vi "Add_Update_Values_sub.vi"(5 "Raw data Filename column name":string, 6 "Edit all Rows?":bool, 7 "Value  Constant?":bool, 8 "Selected Rows":i32[](array[numeric]), 9 "New Values In":string[][](array[string]), 10 "New Chs In":string[](array[string])=[""], 11 "Filename":path) -> (1 "Edit Info":string[][](array[string]))   [LabVIEW 2010]
uses:
  Globals/Constants_global.vi
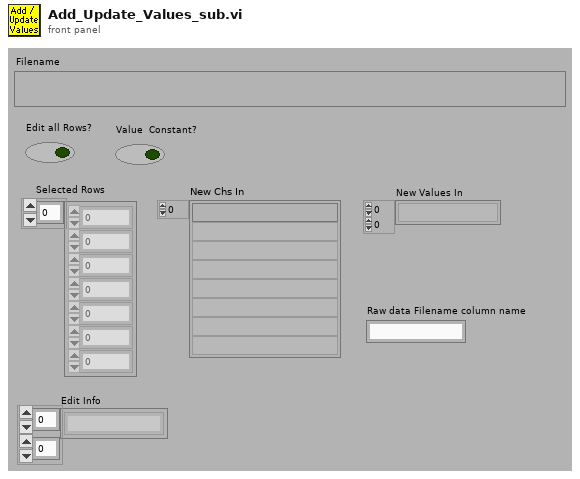
[diagram p1: front panel]
types:
  T1 = enum16{"read/write", "read-only", "write-only", "write-only (truncate)"}
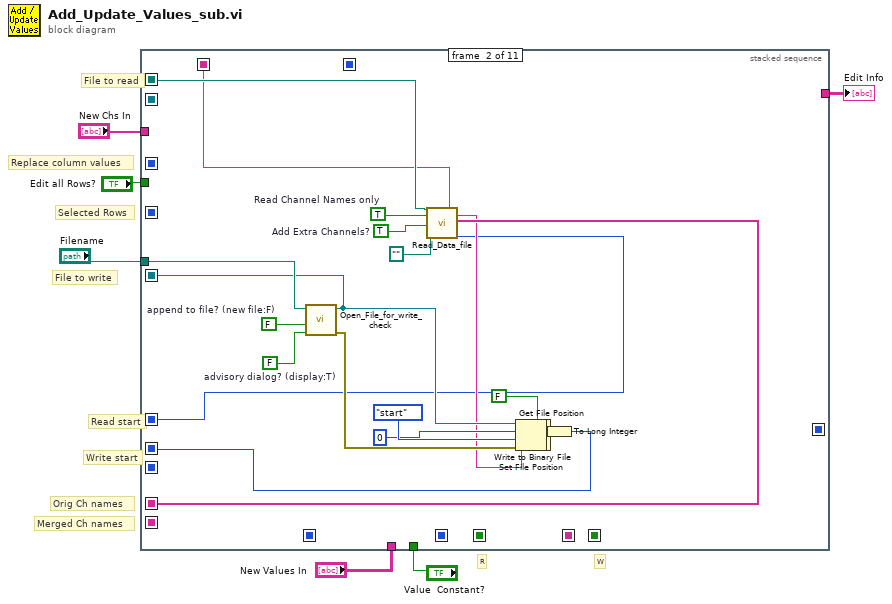
[diagram p0: block diagram]
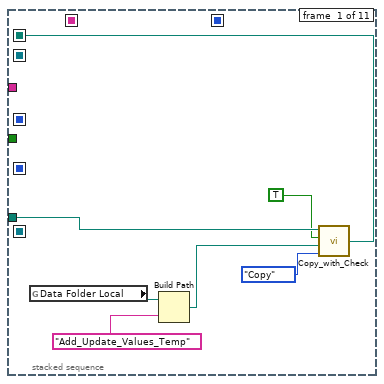
[diagram p2: hidden frame]
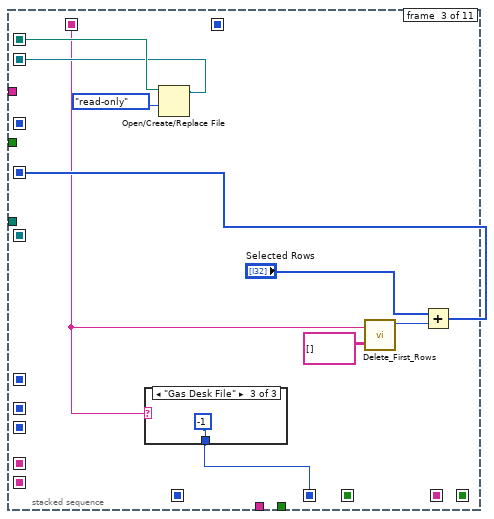
[diagram p3: hidden frame]
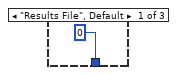
[diagram p4: hidden frame]
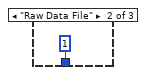
[diagram p5: hidden frame]
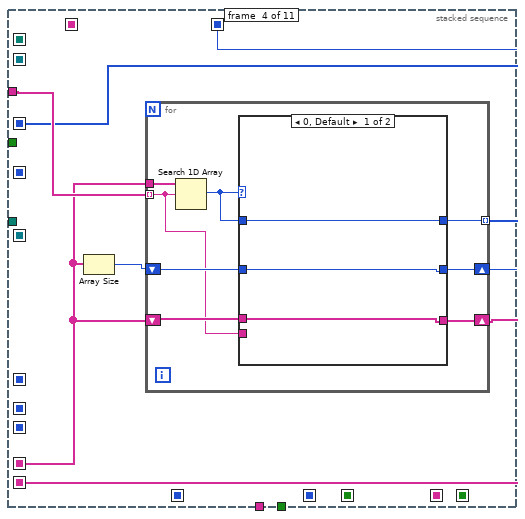
[diagram p6: hidden frame]
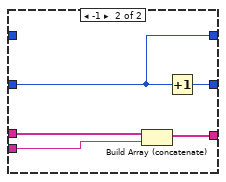
[diagram p7: hidden frame]
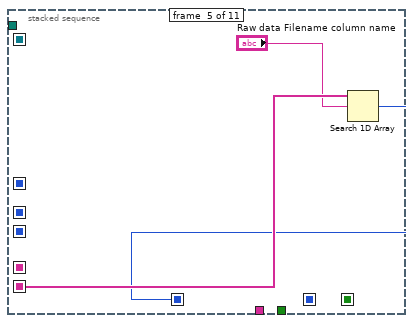
[diagram p8: hidden frame]
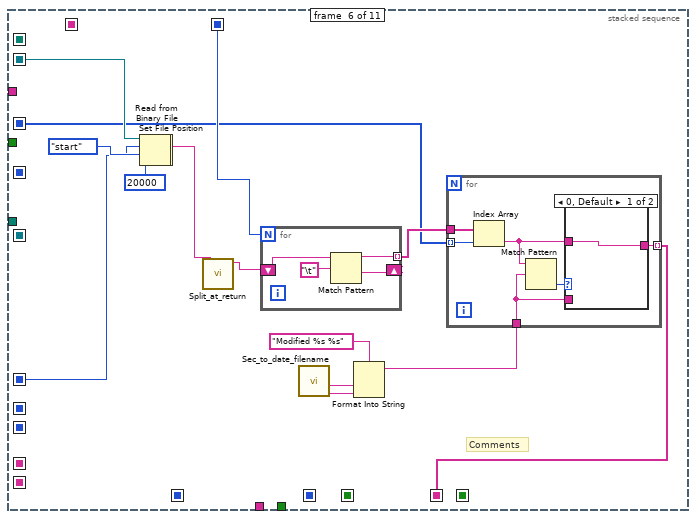
[diagram p9: hidden frame]
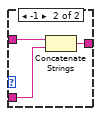
[diagram p10: hidden frame]
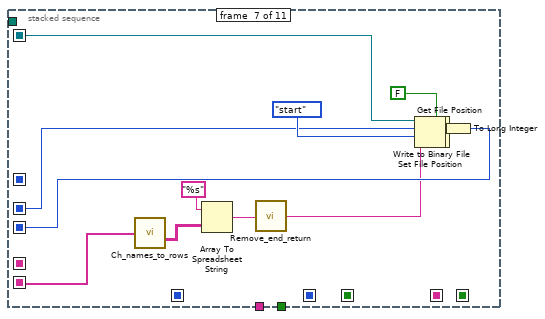
[diagram p11: hidden frame]
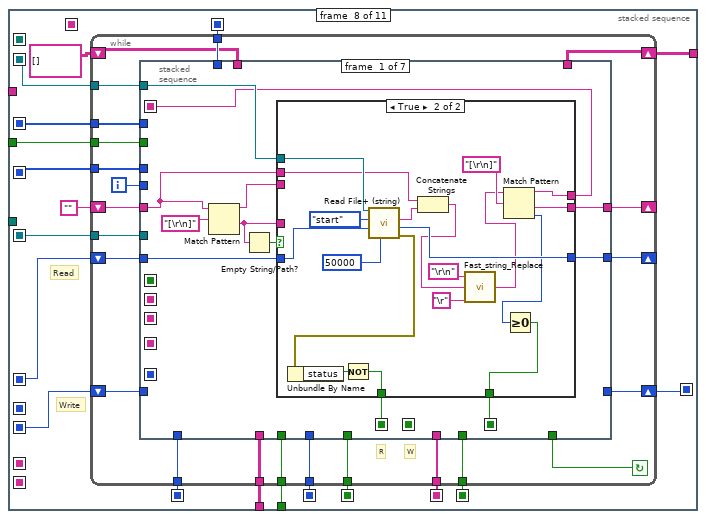
[diagram p12: hidden frame]
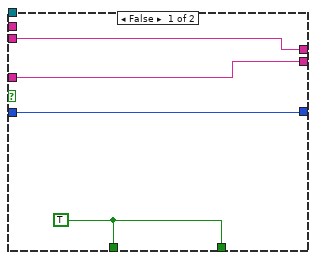
[diagram p13: hidden frame]
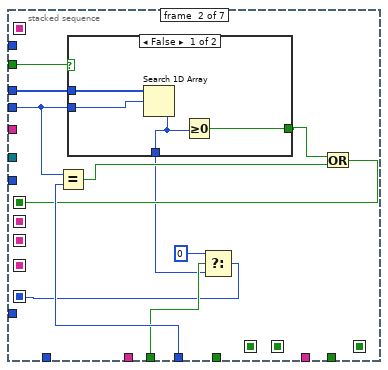
[diagram p14: hidden frame]
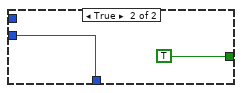
[diagram p15: hidden frame]
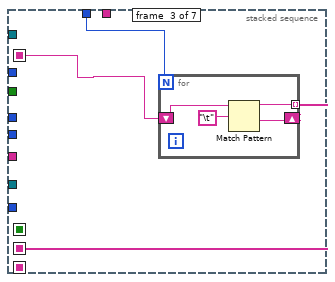
[diagram p16: hidden frame]
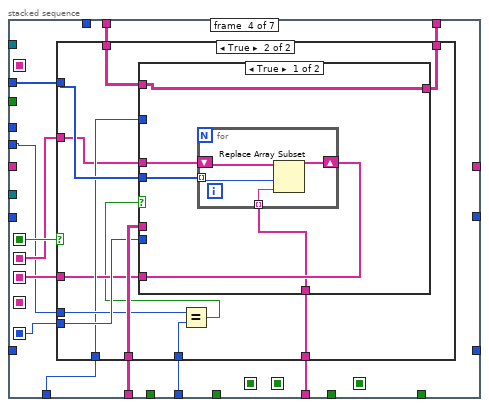
[diagram p17: hidden frame]
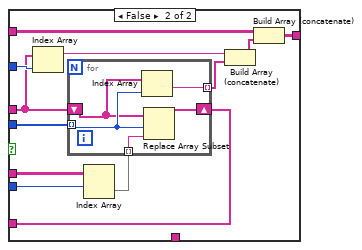
[diagram p19: hidden frame]
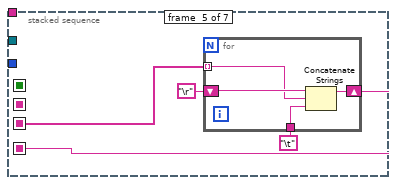
[diagram p20: hidden frame]
diagram:
  # "File to read"
  # "File to write"
  # "Merged Ch names"
  # "Orig Ch names"
  # "Replace column values"
  # "Selected Rows"
  # "Read start"
  # "Write start"
  # "W"
  # "R"
  n1 = stacked-sequence {
    seq-local: [_ _ w39 _ _ _ _ _ _ _ _] -> [_ _ _ _ _ w86 _ w129 _ w306 _]
    seq-local: [_ w22 _ _ _ _ _ _ _ _ _] -> [_ _ _ _ _ w85 _ w131 _ _ _]
    seq-local: [_ _ _ _ _ _ _ w135 _ _ _] -> [_ _ _ _ _ _ _ _ _ _ w310]
    seq-local: [_ _ _ _ _ _ _ w134 _ _ _] -> [_ _ _ _ _ _ _ _ _ _ w312]
    seq-local: [_ _ _ _ _ _ _ w133 _ _ _] -> [_ _ _ _ _ _ _ _ w303 _ _]
    seq-local: [_ _ w42 _ _ _ _ _ _ _ _] -> [_ _ _ _ _ _ _ w132 _ _ _]
    seq-local: [_ w23 _ _ _ _ _ _ _ _ _] -> [_ _ _ _ _ _ w111 _ _ _ _]
    seq-local: [_ w33 _ _ _ _ _ _ _ _ _] -> [_ _ _ w50 _ _ _ _ _ _ _]
    seq-local: [_ _ _ w51 _ _ _ _ _ _ _] -> [_ _ _ _ _ w80 _ w127 _ _ _]
    seq-local: [_ w25 _ _ _ _ _ _ _ _ _] -> [_ _ _ _ _ _ w112 w130 w301 w304 _]
    seq-local: [_ _ _ w49 _ _ _ _ _ _ _] -> [_ _ _ _ _ w88 _ w128 _ _ _]
    seq-local: [_ _ _ w48 _ _ _ _ _ _ _] -> [_ _ _ _ w72 _ w115 _ _ _ _]
    seq-local: [w8 _ _ _ _ _ _ _ _ _ _] -> [_ w32 w40 _ _ _ _ _ _ _ w308]
    seq-local: [_ _ _ _ _ _ w110 _ _ _ _] -> [_ _ _ _ _ _ _ w126 _ _ _]
    seq-local: [_ w21 _ _ _ _ _ _ _ _ _] -> [_ _ w37 _ _ _ _ _ _ _ _]
    seq-local: [_ _ _ _ _ w76 _ _ _ _ _] -> [_ _ _ _ _ _ _ w121 _ _ _]
    seq-local: [_ _ w38 _ _ _ _ _ _ _ _] -> [_ _ _ _ _ _ _ w122 _ _ _]
    seq-local: [_ _ _ _ w71 _ _ _ _ _ _] -> [_ _ _ _ _ _ _ w120 _ _ _]
    tunnel: "Filename" -> [w10 w26 _ _ _ _ _ _ _ _ w309]
    tunnel: "New Chs In" -> [_ _ _ w53 _ _ _ _ _ _ _]
    tunnel: "Edit all Rows?" -> [_ _ _ _ _ _ _ w125 _ _ _]
    tunnel: "New Values In" -> [_ _ _ _ _ _ _ w124 _ _ _]
    tunnel: "Value  Constant?" -> [_ _ _ _ _ _ _ w123 _ _ _]
    tunnel: [_ _ _ _ _ _ _ w118 _ _ _] -> w1
    frame #0 {
      n2 = global read "Constants_global.vi" "Data Folder Local"() -> (w12:path)
      n3 = Build Path(base path=w12, name or relative path="Add_Update_Values_Temp") -> (appended path=w11:path)
      n4 = call "Copy_with_Check.vi"("Mode"=enum16{"Move", "Copy"}."Copy", "Target Path"=w11, "Variable Target?"=TRUE, "Source Path"=w10) -> ("Pathname Out"=w8:path)
    }
    frame #1 {
      w14 = TRUE  # Add Extra Channels?
      w30 = FALSE  # advisory dialog? (display:T)
      w31 = FALSE  # append to file? (new file:F)
      w34 = TRUE  # Read Channel Names only
      n5 = call "Open_File_for_write_check.vi"("advisory dialog? (display:T)"=w30, "append to file? (new file:F)"=w31, "file path"=w26) -> ("error out"=w27:errorcluster, "refnum"=w25:refnum<file>)  [unwired: 7 out]
      n6 = call "Read_Data_file.vi"("Results file"=w32, "Read Channel Names only"=w34, "Add Extra Channels?"=w14, "Template File"=path "") -> ("Filetype"=w21:string, "String Before"=w24:string, "Ch names Out"=w33:string[], "mark after read (chars.)"=w22:i32)  [unwired: 1 in, 11 out]
      n7 = Set File Position(offset (in bytes) (0)=0 ("pos offset (0)"), refnum=w25, from (0:start)=enum16{"start", "end", "current"}."start" ("pos mode (0:2)"), error in=w27) -> (refnum out=w20:refnum<file>, error out=w19:errorcluster)
      n8 = Write to Binary File(file (use dialog)=w20, data=w24, error in=w19, 5:FALSE ("prepend array or string size? (T)")) -> (refnum out=w18:refnum<file>, error out=w17:errorcluster)  [unwired: 3 out]
      n9 = Get File Position(4:w17, 7:w18) -> (2:w16:i64)  [unwired: 2 out]
      n10 = To Long Integer(number=w16) -> (32bit integer=w23:i32)
    }
    frame #2 {
      n11 = case shown="\"Gas Desk File\"" w37 {
        tunnel: [0 ("Comments Row Number") 1 ("Comments Row Number") -1 ("Comments Row Number")] -> w38
        frame "Results File", Default {
        }
        frame "Raw Data File" {
        }
        frame "Gas Desk File" {
        }
      }
      n12 = Open/Create/Replace File(file path (use dialog)=w40, access (0:read/write)=T1."read-only" ("open mode (0)")) -> (refnum out=w39:refnum<file>)  [unwired: 1 in, 5 out]
      n13 = call "Delete_First_Rows.vi"("Data In"=string[][] [], "File Type"=w37) -> ("Rows removed"=w44:i32)  [unwired: 1 out]
      n14 = Add(x="Selected Rows", y=w44) -> (x+y=w42:i32[])
    }
    frame #3 {
      n15 = Array Size(array=w50) -> (size(s)=w52:i32)
      n16 = for {
        tunnel: w50 -> [w61]
        tunnel: w53 -> [w54] mode=indexing
        shift-right: [w60] -> w49
        shift-left: w52 -> [w59]
        tunnel: [w58] -> w51 mode=indexing
        shift-right: [w55] -> w48
        shift-left: w50 -> [w56]
        n17 = Search 1D Array(1D array=w61, element=w54) -> (index of element=w57:i32)  [unwired: 1 out]
        n18 = case shown="0, Default" w57 {
          tunnel: [w63 w69] -> w60
          tunnel: w59 -> [w63 w68]
          tunnel: [w64 w68] -> w58
          tunnel: w57 -> [w64 _]
          tunnel: w56 -> [w62 w67]
          tunnel: [w62 w66] -> w55
          tunnel: w54 -> [_ w65]
          frame 0, Default {
          }
          frame -1 {
            n19 = Build Array (concatenate)(w67, w65) -> (w66:string[])
            n20 = Increment(x=w68) -> (x+1=w69:i32)
          }
        }
      }
    }
    frame #4 {
      n21 = Search 1D Array(1D array=w72, element="Raw data Filename column name") -> (index of element=w71:i32)  [unwired: 1 out]
    }
    frame #5 {
      # "Comments"
      n22 = Set File Position(offset (in bytes) (0)=w85, refnum=w86, from (0:start)=enum16{"start", "end", "current"}."start" ("pos mode (rel. to current:2)")) -> (refnum out=w74:refnum<file>, error out=w73:errorcluster)  [unwired: 1 in]
      n23 = Read from Binary File(8:w73, 10:20000 ("count"), 11:w74) -> (2:w83:string)  [unwired: 6 out]
      n24 = call "Split_at_return.vi"("String"=w83) -> ("before substring"=w82:string)  [unwired: 1 in, 3 out]
      n25 = for {
        N: w88 -> [_]
        shift-right: [w100] -> _
        shift-left: w82 -> [w101]
        tunnel: [w99] -> w81 mode=indexing
        n26 = Match Pattern(string=w101, regular expression="\t") -> (before substring=w99:string, after substring=w100:string)  [unwired: 3 out]
      }
      n27 = call "Sec_to_date_filename.vi"() -> ("Day"=w78:string, "Time"=w75:string)  [unwired: 1 in, 2 out]
      n28 = Format Into String(format string="Modified %s %s" ("Format String"), w78, w75) -> (resulting string=w77:string)  [unwired: 2 in, 1 out]
      n29 = for {
        tunnel: w81 -> [w94]
        tunnel: w80 -> [w93] mode=indexing
        tunnel: w77 -> [w91]
        tunnel: [w92] -> w76 mode=indexing
        n30 = Index Array(array=w94, index=w93) -> (element=w90:string)
        n31 = Match Pattern(string=w90, regular expression=w91) -> (offset past match=w89:i32)  [unwired: 4 out]
        n32 = case shown="0, Default" w89 {
          tunnel: w90 -> [w95 w98]
          tunnel: w91 -> [_ w97]
          tunnel: [w95 w96] -> w92
          frame 0, Default {
          }
          frame -1 {
            n33 = Concatenate Strings(w98, w97) -> (w96:string)
          }
        }
      }
    }
    frame #6 {
      n34 = call "Ch_names_to_rows.vi"("Channel Names"=w115) -> ("3 Row names"=w116:string[][])
      n35 = Array To Spreadsheet String(array=w116, 3:"%s" ("format string")) -> (spreadsheet string=w114:string)  [unwired: 1 out]
      n36 = call "Remove_end_return.vi"("Input string"=w114) -> ("Output string"=w109:string)
      n37 = Set File Position(offset (in bytes) (0)=w111, refnum=w112, from (0:start)=enum16{"start", "end", "current"}."start" ("pos mode (0:2)")) -> (refnum out=w108:refnum<file>, error out=w107:errorcluster)  [unwired: 1 in]
      n38 = Write to Binary File(file (use dialog)=w108, data=w109, error in=w107, 5:FALSE ("prepend array or string size? (T)")) -> (refnum out=w106:refnum<file>, error out=w105:errorcluster)  [unwired: 3 out]
      n39 = Get File Position(4:w105, 7:w106) -> (2:w104:i64)  [unwired: 2 out]
      n40 = To Long Integer(number=w104) -> (32bit integer=w110:i32)
    }
    frame #7 {
      # "Write"
      # "Read"
      n41 = while {
        tunnel: [w150] -> w134
        tunnel: [w151] -> w135
        shift-left: w126 -> [w154]
        shift-right: [w153] -> w133
        tunnel: w129 -> [w156]
        shift-left: w131 -> [w158]
        shift-right: [w157] -> _
        shift-left: "" -> [w159]
        shift-right: [w155] -> _
        tunnel: w132 -> [w149]
        tunnel: w130 -> [w147]
        tunnel: w128 -> [w146]
        tunnel: w125 -> [w145]
        tunnel: w127 -> [w144]
        tunnel: w124 -> [w143]
        tunnel: w123 -> [w142]
        tunnel: w122 -> [w141]
        tunnel: w121 -> [w140]
        tunnel: w120 -> [w139]
        shift-right: [w137] -> w118
        shift-left: string[][] [] -> [w138]
        i -> [w148]
        stop <- w152 continue-if-true
        # "R"
        # "W"
        n42 = stacked-sequence {
          seq-local: [w165 _ _ _ _ _ _] -> [_ _ w213 _ _ _ _]
          seq-local: [_ _ _ _ _ w291 _] -> [_ _ _ _ _ _ w294]
          seq-local: [w166 _ _ _ _ _ _] -> [_ _ _ _ _ _ w296]
          seq-local: [w167 _ _ _ _ _ _] -> [_ _ _ _ _ _ w295]
          seq-local: [_ w200 _ _ _ _ _] -> [_ _ _ w229 _ _ _]
          seq-local: [_ _ _ _ w274 _ _] -> [_ _ _ _ _ w290 _]
          seq-local: [_ _ w212 _ _ _ _] -> [_ _ _ w227 _ _ _]
          seq-local: [_ _ _ w226 _ _ _] -> [_ _ _ _ w271 _ _]
          seq-local: [_ w195 _ _ _ _ _] -> [_ _ _ w219 _ _ _]
          tunnel: w159 -> [w163 _ _ _ _ _ _]
          tunnel: w158 -> [w171 _ _ _ _ _ _]
          tunnel: [w170 _ _ _ _ _ _] -> w157
          tunnel: w156 -> [w169 _ _ _ _ _ _]
          tunnel: [w168 _ _ _ _ _ _] -> w155
          tunnel: w154 -> [_ _ _ _ _ w293 _]
          tunnel: [_ _ _ _ _ w292 _] -> w153
          tunnel: [_ _ _ _ _ _ w297] -> w152
          tunnel: [_ _ _ _ _ _ w295] -> w151
          tunnel: [_ _ _ _ _ _ w294] -> w150
          tunnel: w149 -> [_ w205 _ _ _ _ _]
          tunnel: w148 -> [_ w202 _ w224 _ _ _]
          tunnel: w147 -> [_ _ _ _ _ w289 _]
          tunnel: w146 -> [_ _ w214 _ _ _ _]
          tunnel: w145 -> [_ w204 _ _ _ _ _]
          tunnel: w144 -> [_ _ _ w230 _ _ _]
          tunnel: w143 -> [_ _ _ w228 _ _ _]
          tunnel: w142 -> [_ w198 _ _ _ _ _]
          tunnel: w141 -> [_ w203 _ w225 _ _ _]
          tunnel: w140 -> [_ _ _ w223 _ _ _]
          tunnel: w139 -> [_ _ _ w222 _ _ _]
          tunnel: w138 -> [_ _ _ w221 _ _ _]
          tunnel: [_ _ _ w220 _ _ _] -> w137
          frame #0 {
            n43 = Match Pattern(string=w163, regular expression="[\r\n]") -> (before substring=w162:string, after substring=w160:string)  [unwired: 3 out]
            n44 = Empty String/Path?(string/path=w160) -> (empty?=w161:bool)
            n45 = case shown="True" w161 {
              tunnel: w171 -> [w175 w194]
              tunnel: [w175 w192] -> w170
              tunnel: w169 -> [_ w191]
              tunnel: w163 -> [_ w190]
              tunnel: [w174 w182] -> w168
              tunnel: w160 -> [w174 _]
              tunnel: [w173 w187] -> w167
              tunnel: [w173 w179] -> w166
              tunnel: [w172 w181] -> w165
              tunnel: w162 -> [w172 _]
              frame False {
                w173 = TRUE
              }
              frame True {
                n46 = call <vilib>:"Read File+ (string).vi"("count"=50000, "pos offset (bytes:0)"=w194, "pos mode (rel. to current:2)"=enum16{"start", "end", "current"}."start", "refnum"=w191) -> ("error out"=w189:errorcluster, "mark after read (bytes)"=w192:i32, "string"=w178:string)  [unwired: 1 in, 4 out]
                n47 = Unbundle By Name(w189) -> ("status"=w188:bool)
                n48 = Not(x=w188) -> (.not. x?=w187:bool)
                n49 = Concatenate Strings(w190, w178) -> (w177:string)
                n50 = call "Fast_string_Replace.vi"("Replace match with:"="\r" ("regular expression"), "Input String"=w177, "regular expression"="\r\n") -> ("Output String"=w176:string)  [unwired: 2 out]
                n51 = Match Pattern(string=w176, regular expression="[\r\n]") -> (before substring=w181:string, after substring=w182:string, offset past match=w180:i32)  [unwired: 2 out]
                n52 = Greater Or Equal To 0?(x=w180) -> (x >= 0?=w179:bool)
              }
            }
          }
          frame #1 {
            n53 = Equal?(x=w202, y=w203) -> (x = y?=w201:bool)
            n54 = case shown="False" w204 {
              tunnel: w205 -> [w209 _]
              tunnel: w202 -> [w208 w210]
              tunnel: [w207 TRUE] -> w199
              tunnel: [w206 w210] -> w197
              frame False {
                n55 = Search 1D Array(1D array=w209, element=w208) -> (index of element=w206:i32)  [unwired: 1 out]
                n56 = Greater Or Equal To 0?(x=w206) -> (x >= 0?=w207:bool)
              }
              frame True {
              }
            }
            n57 = Select(t=0, s=w198, f=w197) -> (s? t:f=w195:i32)
            n58 = Or(x=w199, y=w201) -> (x .or. y?=w200:bool)
          }
          frame #2 {
            n59 = for {
              N: w214 -> [_]
              shift-right: [w216] -> _
              shift-left: w213 -> [w217]
              tunnel: [w215] -> w212 mode=indexing
              n60 = Match Pattern(string=w217, regular expression="\t") -> (before substring=w215:string, after substring=w216:string)  [unwired: 3 out]
            }
          }
          frame #3 {
            n61 = case shown="True" w229 {
              tunnel: w230 -> [_ w244]
              tunnel: w228 -> [_ w243]
              tunnel: w227 -> [w232 w237]
              tunnel: w219 -> [_ w242]
              tunnel: [w232 w238] -> w226
              tunnel: w225 -> [_ w241]
              tunnel: w224 -> [_ w240]
              tunnel: w223 -> [_ w233]
              tunnel: w222 -> [_ w239]
              tunnel: w221 -> [w231 w236]
              tunnel: [w231 w235] -> w220
              frame False {
              }
              frame True {
                n62 = Equal?(x=w240, y=w241) -> (x = y?=w234:bool)
                n63 = case shown="True" w234 {
                  tunnel: w244 -> [w249 w265]
                  tunnel: w243 -> [_ w264]
                  tunnel: w242 -> [_ w263]
                  tunnel: w239 -> [_ w261]
                  tunnel: [w248 w260] -> w238
                  tunnel: w237 -> [w247 w254]
                  tunnel: w236 -> [w245 w259]
                  tunnel: [w245 w258] -> w235
                  tunnel: w233 -> [w246 _]
                  frame True {
                    n64 = for {
                      shift-right: [w253] -> w248
                      shift-left: w247 -> [w251]
                      tunnel: w249 -> [w252] mode=indexing
                      tunnel: w246 -> [w250] mode=indexing
                      n65 = Replace Array Subset(array=w251, new element=w250, index=w252) -> (w253:string[])
                    }
                  }
                  frame False {
                    n66 = Index Array(array=w254, index=w261) -> (element=w256:string)
                    n67 = Index Array(array=w264, index (row)=w263) -> (element=w262:string[])  [unwired: 1 in]
                    n68 = for {
                      shift-right: [w270] -> w260
                      shift-left: w254 -> [w268]
                      tunnel: w265 -> [w269] mode=indexing
                      tunnel: w262 -> [w267] mode=indexing
                      tunnel: [w266] -> w257 mode=indexing
                      n69 = Index Array(array=w268, index=w269) -> (element=w266:string)
                      n70 = Replace Array Subset(array=w268, new element=w267, index=w269) -> (w270:string[])
                    }
                    n71 = Build Array (concatenate)(w256, w257) -> (w255:string[])
                    n72 = Build Array (concatenate)(w259, w255) -> (w258:string[][])
                  }
                }
              }
            }
          }
          frame #4 {
            n73 = for {
              tunnel: w271 -> [w275] mode=indexing
              shift-right: [w276] -> w274
              shift-left: "\r" -> [w278]
              tunnel: "\t" -> [w277]
              n74 = Concatenate Strings(w278, w275, w277) -> (w276:string)
            }
          }
          frame #5 {
            n75 = Set File Position(offset (in bytes) (0)=w293, refnum=w289, from (0:start)=enum16{"start", "end", "current"}."start" ("pos mode (0:2)")) -> (refnum out=w284:refnum<file>, error out=w283:errorcluster)  [unwired: 1 in]
            n76 = Write to Binary File(file (use dialog)=w284, data=w290, error in=w283, 5:FALSE ("prepend array or string size? (T)")) -> (refnum out=w282:refnum<file>, error out=w281:errorcluster)  [unwired: 3 out]
            n77 = Get File Position(4:w281, 7:w282) -> (0:w285:errorcluster, 2:w280:i64)  [unwired: 1 out]
            n78 = Unbundle By Name(w285) -> ("status"=w286:bool)
            n79 = To Long Integer(number=w280) -> (32bit integer=w288:i32)
            n80 = Decrement(x=w288) -> (x-1=w292:i32)
            n81 = Not(x=w286) -> (.not. x?=w291:bool)
          }
          frame #6 {
            n82 = Compound Arithmetic op=AND(w295, w294, w296) -> (w297:bool)
          }
        }
      }
    }
    frame #8 {
      n83 = call <vilib>:"compatCalcOffset.vi"("pos offset (0)"=w303, "pos mode (0:1)"=enum16{"start", "end", "current"}."start", "refnum"=w301) -> ("error out"=w300:errorcluster, "offset"=w299:i32, "dup refnum"=w298:refnum<file>)  [unwired: 1 in, 5 out]
      n84 = Set File Size(4:w300, 6:w299, 7:w298) -> ()  [unwired: 2 out]
    }
    frame #9 {
      n85 = Build Array(w306, w304) -> (w305:refnum<file>[])
      n86 = for {
        tunnel: w305 -> [w307] mode=indexing
        n87 = Close File(refnum=w307) -> ()  [unwired: 1 in, 2 out]
      }
    }
    frame #10 {
      n88 = Not And(1:w312, 2:w310) -> (0:w311:bool)
      n89 = case shown="True" w311 {
        tunnel: w308 -> [_ w315]
        tunnel: w309 -> [_ w314]
        frame False {
        }
        frame True {
          w319 = TRUE  # Dialog Box
          n90 = Format Into String(format string="whilst reading from file %s\nand writing to file %s", w315, w314) -> (resulting string=w313:string)  [unwired: 2 in, 1 out]
          n91 = Bundle By Name(cluster=errorcluster {"status"=FALSE, "code"=0, "source"=""} ("error in (no error)"), "status"=TRUE ("Bundle Element"), "source"=w313) -> (w320:errorcluster)
          n92 = call "EnFlo_Error_Handler.vi"("error in (no error)"=w320, "Error Type"="File Rewrite Error", "Dialog Box (T)"=w319) -> ()  [unwired: 3 out]
        }
      }
    }
  }
  "Edit Info" <- w1
